vi "LS Das Bank2 Error Index.vi"(0 "RowCountSlow":i32, 5 "SlowRecordIndexes":i32[](array[numeric]), 7 "Bank2SlowRecord":bool, 9 "RowCountStandard":i32, 11 "ErrorIndex":i32) -> (4 "Bank2ErrorIndex":string)   [LabVIEW 2013]
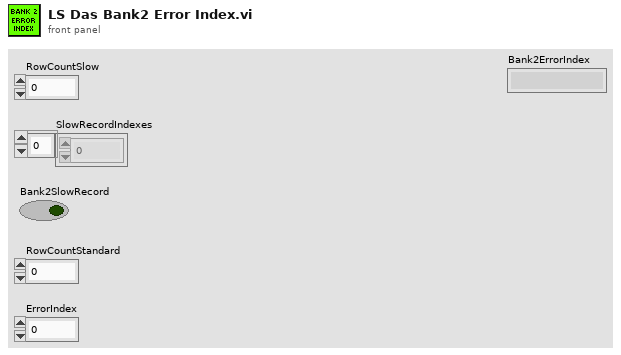
[diagram p1: front panel]
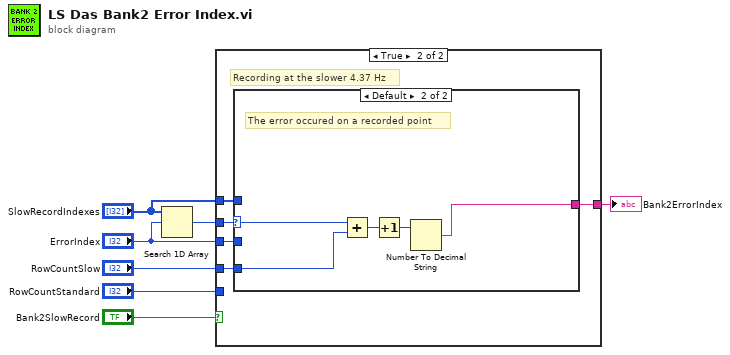
[diagram p0: block diagram]
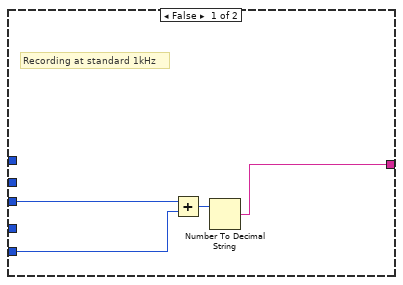
[diagram p2: hidden frame]
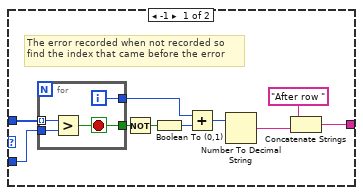
[diagram p3: hidden frame]
diagram:
  n1 = Search 1D Array(1D array="SlowRecordIndexes", element="ErrorIndex") -> (index of element=w7:i32)  [unwired: 1 in]
  n2 = case shown="True" "Bank2SlowRecord" {
    tunnel: w7 -> [_ w16]
    tunnel: "RowCountSlow" -> [_ w15]
    tunnel: "SlowRecordIndexes" -> [_ w14]
    tunnel: "ErrorIndex" -> [w10 w13]
    tunnel: "RowCountStandard" -> [w11 _]
    tunnel: [w8 w12] -> w1
    frame False {
      # "Recording at standard 1kHz"
      n3 = Add(x=w10, y=w11) -> (x+y=w9:i32)
      n4 = Number To Decimal String(number=w9) -> (decimal integer string=w8:string)  [unwired: 1 in]
    }
    frame True {
      # "Recording at the slower 4.37 Hz"
      n5 = case shown="Default" w16 {
        selector: w16 -> [_ w35]
        tunnel: w15 -> [_ w34]
        tunnel: w14 -> [w26 _]
        tunnel: w13 -> [w25 _]
        tunnel: [w17 w31] -> w12
        frame -1 {
          # "The error recorded when not recorded so\nfind the index that came before the error"
          n6 = for {
            tunnel: w26 -> [w30] mode=indexing
            tunnel: w25 -> [w29]
            tunnel: [w28] -> w21
            tunnel: [w27] -> w24
            i -> [w28]
            stop <- w27 stop-if-true
            n7 = Greater?(x=w30, y=w29) -> (0:w27:bool)
          }
          n8 = Not(x=w24) -> (.not. x?=w23:bool)
          n9 = Boolean To (0,1)(Boolean=w23) -> (0, 1=w22:i16)
          n10 = Add(x=w21, y=w22) -> (x+y=w20:i32)
          n11 = Number To Decimal String(number=w20) -> (decimal integer string=w18:string)  [unwired: 1 in]
          n12 = Concatenate Strings("After row ", w18) -> (w17:string)
        }
        frame Default {
          # "The error occured on a recorded point"
          n13 = Add(x=w35, y=w34) -> (x+y=w33:i32)
          n14 = Increment(x=w33) -> (x+1=w32:i32)
          n15 = Number To Decimal String(number=w32) -> (decimal integer string=w31:string)  [unwired: 1 in]
        }
      }
    }
  }
  "Bank2ErrorIndex" <- w1
